vi "DAC Save Results.vi"(8 "error in":errorcluster, 9 "Log Details?":bool, 10 "tdms file":refnum<k34>, 11 "DAC FTCU in":refnum<class "DAC FTCU.lvclass">) -> (0 "error out":errorcluster)   [LabVIEW 2019, in "DAC.lvlib" / "DAC FTCU.lvclass"]
uses:
  DAC FTCU.lvclass
  C:/Users/wg/Documents/LV_Projects/test-stand/App/DAC/DAC.lvclass
  DAC.lvclass/DAC.ctl
  DAC FTCU.lvclass/DAC FTCU.ctl
  DAC.lvclass
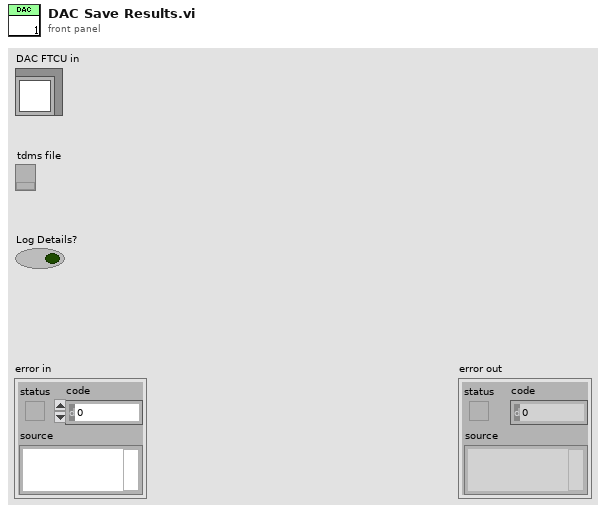
[diagram p1: front panel]
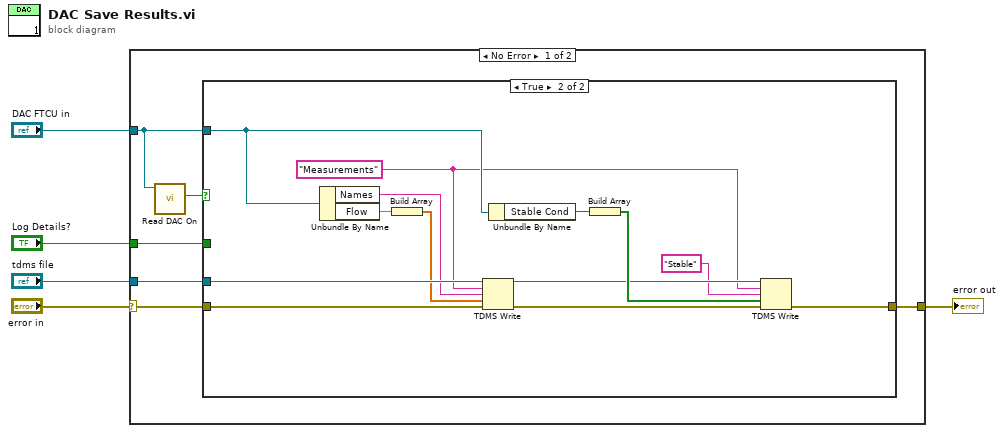
[diagram p0: block diagram]
diagram:
  n1 = case shown="No Error" "error in" {
    selector: "error in" -> [w8 w26]
    tunnel: "DAC FTCU in" -> [w11 _]
    tunnel: "tdms file" -> [w9 _]
    tunnel: [w7 w26] -> w2
    tunnel: "Log Details?" -> [w6 _]
    frame No Error {
      n2 = call "Read DAC On.vi"("DAC in"=w11) -> ("DAC On"=w10:bool)  [unwired: 8 in, 2 out]
      n3 = case shown="True" w10 {
        tunnel: w11 -> [_ w20]
        tunnel: w9 -> [_ w25]
        tunnel: w8 -> [w12 w24]
        tunnel: [w12 w16] -> w7
        tunnel: w6 -> [_ _]
        frame False {
        }
        frame True {
          w14 = "Measurements" ("group name in (Untitled)")
          n4 = Unbundle By Name(w20) -> ("Names"=w21:string, "Flow"=w23:sgl)
          n5 = Build Array(w23) -> (w22:sgl[])
          n6 = TDMS Write(0:w25, 5:w14, 7:w21, 9:w22, 11:w24) -> (4:w15:refnum<k34>, 15:w17:errorcluster)  [unwired: 1 in, 2 out]
          n7 = Unbundle By Name(w20) -> ("Stable Cond"=w19:bool)
          n8 = Build Array(w19) -> (w18:bool[])
          n9 = TDMS Write(0:w15, 5:w14, 7:"Stable" ("delimiter"), 9:w18, 11:w17) -> (15:w16:errorcluster)  [unwired: 1 in, 3 out]
        }
      }
    }
    frame Error {
    }
  }
  "error out" <- w2
